vi "Verify Test.vi"(0 "Test Parameters In":string[][](table) caption="Parameter Information", 7 "Brushed?":bool, 9 "Maxes":dbl[](array[numeric]), 11 "Mins":dbl[](array[numeric])) -> (4 "Test Parameters Out":string[][](table) caption="Parameter Information", 8 "Altered?":bool, 10 "ValidColumns?":bool, 15 "ValidParameters?":bool)   [LabVIEW 2013]
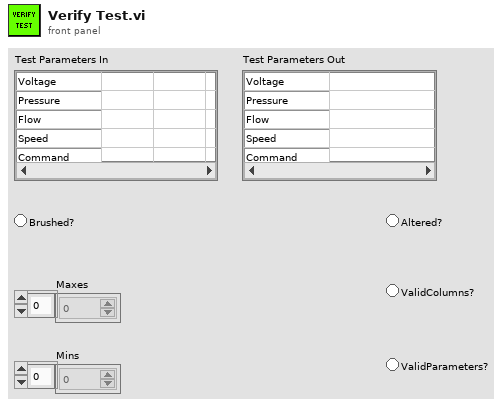
[diagram p1: front panel]
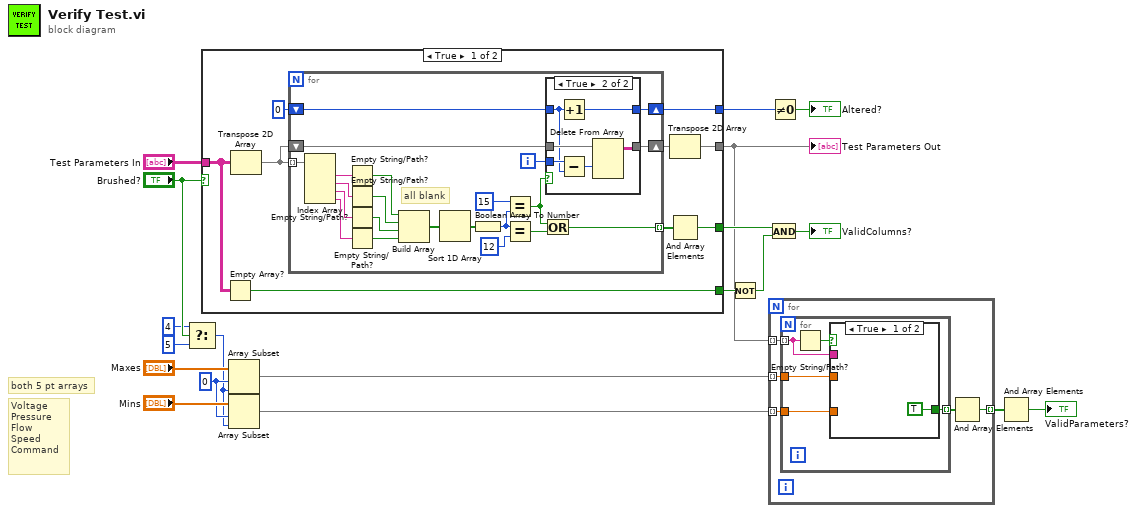
[diagram p0: block diagram]
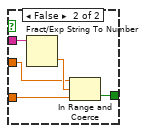
[diagram p2: hidden frame]
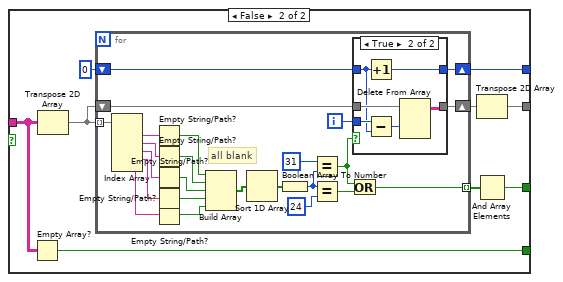
[diagram p4: hidden frame]
diagram:
  w10 = 0 ("index")
  # "Voltage\nPressure\nFlow\nSpeed\nCommand"
  # "both 5 pt arrays"
  n1 = Select(t=4 ("length"), s="Brushed?", f=5 ("length")) -> (s? t:f=w6:i32)
  n2 = case shown="True" "Brushed?" {
    tunnel: [w23 w62] -> w15
    tunnel: [w25 w64] -> w18
    tunnel: [w22 w61] -> w16
    tunnel: "Test Parameters In" -> [w21 w60]
    tunnel: [w20 w59] -> w5
    frame True {
      n3 = Empty Array?(array=w21) -> (empty?=w22:bool)
      n4 = Transpose 2D Array(2D array=w21) -> (transposed array=w28:string[][])
      n5 = for {
        tunnel: w28 -> [w50] mode=indexing
        tunnel: [w37] -> w24 mode=indexing
        shift-right: [w33] -> w26
        shift-left: w28 -> [w34]
        shift-right: [w29] -> w25
        shift-left: u32 0 ("x") -> [w31]
        i -> [w30]
        # "all blank"
        n6 = Index Array(array=w50) -> (element #1=w49:string, element #2=w39:string, element #3=w48:string, element #4=w47:string)  [unwired: 4 in]
        n7 = Empty String/Path?(string/path=w49) -> (empty?=w46:bool)
        n8 = Empty String/Path?(string/path=w39) -> (empty?=w45:bool)
        n9 = Empty String/Path?(string/path=w48) -> (empty?=w43:bool)
        n10 = Empty String/Path?(string/path=w47) -> (empty?=w44:bool)
        n11 = Build Array(w46, w45, w43, w44) -> (w42:bool[])
        n12 = Sort 1D Array(array=w42) -> (sorted array=w41:bool[])
        n13 = Boolean Array To Number(Boolean array=w41) -> (number=w36:u32)
        n14 = Equal?(x=u32 15, y=w36) -> (x = y?=w32:bool)
        n15 = Equal?(x=w36, y=u32 12) -> (x = y?=w38:bool)
        n16 = Or(x=w32, y=w38) -> (x .or. y?=w37:bool)
        n17 = case shown="True" w32 {
          tunnel: [w52 w57] -> w33
          tunnel: w34 -> [w52 w58]
          tunnel: w31 -> [w51 w54]
          tunnel: w30 -> [_ w55]
          tunnel: [w51 w53] -> w29
          frame False {
          }
          frame True {
            n18 = Increment(x=w54) -> (x+1=w53:u32)
            n19 = Subtract(x=w55, y=w54) -> (x-y=w56:u32)
            n20 = Delete From Array(array=w58, index (row)=w56) -> (array with subset deleted=w57:string[][])  [unwired: 2 in, 1 out]
          }
        }
      }
      n21 = Transpose 2D Array(2D array=w26) -> (transposed array=w20:string[][])
      n22 = And Array Elements(Boolean array=w24) -> (logical AND=w23:bool)
    }
    frame False {
      n23 = Empty Array?(array=w60) -> (empty?=w61:bool)
      n24 = Transpose 2D Array(2D array=w60) -> (transposed array=w67:string[][])
      n25 = for {
        tunnel: w67 -> [w91] mode=indexing
        tunnel: [w76] -> w63 mode=indexing
        shift-right: [w72] -> w65
        shift-left: w67 -> [w73]
        shift-right: [w68] -> w64
        shift-left: u32 0 ("x") -> [w70]
        i -> [w69]
        # "all blank"
        n26 = Index Array(array=w91) -> (element #1=w90:string, element #2=w78:string, element #3=w89:string, element #4=w88:string, element #5=w80:string)  [unwired: 5 in]
        n27 = Empty String/Path?(string/path=w90) -> (empty?=w87:bool)
        n28 = Empty String/Path?(string/path=w78) -> (empty?=w86:bool)
        n29 = Empty String/Path?(string/path=w89) -> (empty?=w84:bool)
        n30 = Empty String/Path?(string/path=w88) -> (empty?=w85:bool)
        n31 = Empty String/Path?(string/path=w80) -> (empty?=w79:bool)
        n32 = Build Array(w87, w86, w84, w85, w79) -> (w83:bool[])
        n33 = Sort 1D Array(array=w83) -> (sorted array=w82:bool[])
        n34 = Boolean Array To Number(Boolean array=w82) -> (number=w75:u32)
        n35 = Equal?(x=u32 31, y=w75) -> (x = y?=w71:bool)
        n36 = Equal?(x=w75, y=u32 24) -> (x = y?=w77:bool)
        n37 = Or(x=w71, y=w77) -> (x .or. y?=w76:bool)
        n38 = case shown="True" w71 {
          tunnel: [w93 w98] -> w72
          tunnel: w73 -> [w93 w99]
          tunnel: w70 -> [w92 w95]
          tunnel: w69 -> [_ w96]
          tunnel: [w92 w94] -> w68
          frame False {
          }
          frame True {
            n39 = Increment(x=w95) -> (x+1=w94:u32)
            n40 = Subtract(x=w96, y=w95) -> (x-y=w97:u32)
            n41 = Delete From Array(array=w99, index (row)=w97) -> (array with subset deleted=w98:string[][])  [unwired: 2 in, 1 out]
          }
        }
      }
      n42 = Transpose 2D Array(2D array=w65) -> (transposed array=w59:string[][])
      n43 = And Array Elements(Boolean array=w63) -> (logical AND=w62:bool)
    }
  }
  "Test Parameters Out" <- w5
  n44 = Array Subset(array="Maxes", index=w10, length=w6) -> (w4:dbl[])
  n45 = Array Subset(array="Mins", index=w10, length=w6) -> (w3:dbl[])
  n46 = Not(x=w16) -> (.not. x?=w17:bool)
  n47 = And(x=w15, y=w17) -> (x .and. y?=→"ValidColumns?":bool)
  n48 = for {
    tunnel: w5 -> [w104] mode=indexing
    tunnel: w4 -> [w103] mode=indexing
    tunnel: w3 -> [w102] mode=indexing
    tunnel: [w100] -> w2 mode=indexing
    n49 = for {
      tunnel: w104 -> [w108] mode=indexing
      tunnel: w103 -> [w107]
      tunnel: w102 -> [w106]
      tunnel: [w105] -> w101 mode=indexing
      n50 = Empty String/Path?(string/path=w108) -> (empty?=w109:bool)
      n51 = case shown="True" w109 {
        tunnel: w108 -> [_ w115]
        tunnel: w107 -> [_ w113]
        tunnel: w106 -> [_ w112]
        tunnel: [TRUE w111] -> w105
        frame True {
        }
        frame False {
          n52 = Fract/Exp String To Number(string=w115) -> (number=w114:dbl)  [unwired: 3 in, 1 out]
          n53 = In Range and Coerce(upper limit=w113, x=w114, lower limit=w112) -> (In Range?=w111:bool)  [unwired: 1 out]
        }
      }
    }
    n54 = And Array Elements(Boolean array=w101) -> (logical AND=w100:bool)
  }
  n55 = Not Equal To 0?(x=w18) -> (x != 0?=→"Altered?":bool)
  n56 = And Array Elements(Boolean array=w2) -> (logical AND=→"ValidParameters?":bool)
